vi "Read Y_A.vi"(8 "error in (no error)":errorcluster, 11 "reg in":refnum<class "bronkhorst_reg_1.lvclass">) -> (0 "error out":errorcluster, 2 "Y_A":dbl step=1.0, 3 "reg out":refnum<class "bronkhorst_reg_1.lvclass">)   [LabVIEW 2019, in "bronkhorst_reg_1.lvclass"]
uses:
  bronkhorst_reg_1.lvclass
  bronkhorst_reg_1.lvclass/bronkhorst_reg_1.ctl
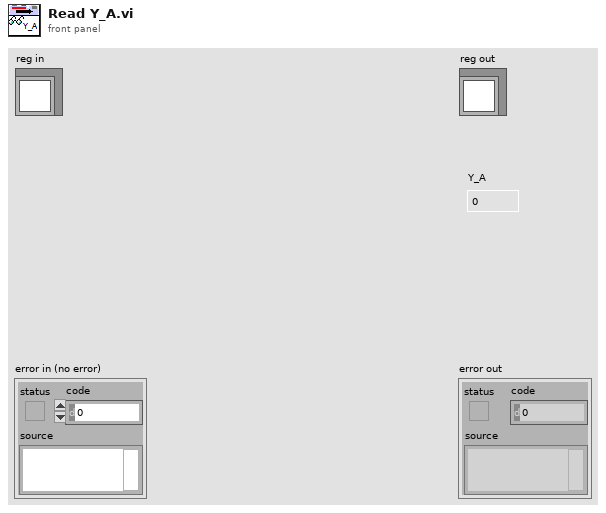
[diagram p1: front panel]
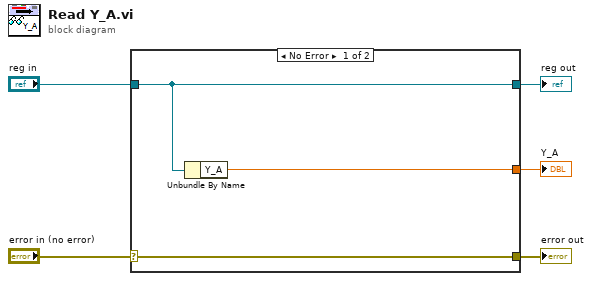
[diagram p0: block diagram]
diagram:
  n1 = case shown="No Error" "error in (no error)" {
    selector: "error in (no error)" -> [w8 w9]
    tunnel: [w8 w9] -> w4
    tunnel: [w7 w10] -> w2
    tunnel: "reg in" -> [w7 w10]
    tunnel: [w6 _] -> w1
    frame No Error {
      n2 = Unbundle By Name(w7) -> ("Y_A"=w6:dbl)
    }
    frame Error {
    }
  }
  "error out" <- w4
  "reg out" <- w2
  "Y_A" <- w1
